vi "Scan Initilize_ver2_2.vi"(0 "VISA Refnum in":refnum<visa-resource-name>, 1 "Scan Measure\nTime":dbl=17.0, 5 "Channel Count":i32, 9 "Current Setting":u8[](array[numeric]), 11 "error in (no error)":errorcluster, 12 "Sample number":i32=1, 13 "Measure Maximun Voltage":dbl=100.0 format="%#_13g", 14 "Enable DMM Relay":bool=TRUE) -> (3 "Current Channel":string[](array[string]), 4 "VISA Refnum out":refnum<visa-resource-name>, 6 "P channel number":i32, 10 "N channel number":i32, 15 "error out":errorcluster)   [LabVIEW 2023]
uses:
  <instrlib>/Agilent 3446X Series/Agilent 3446X Series.lvlib
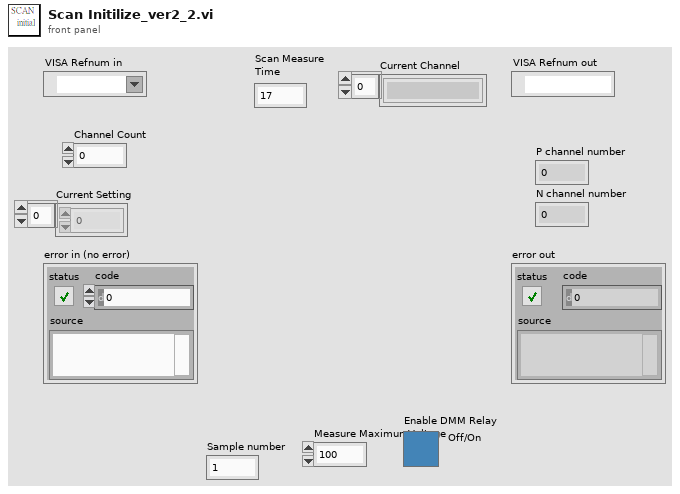
[diagram p1: front panel]
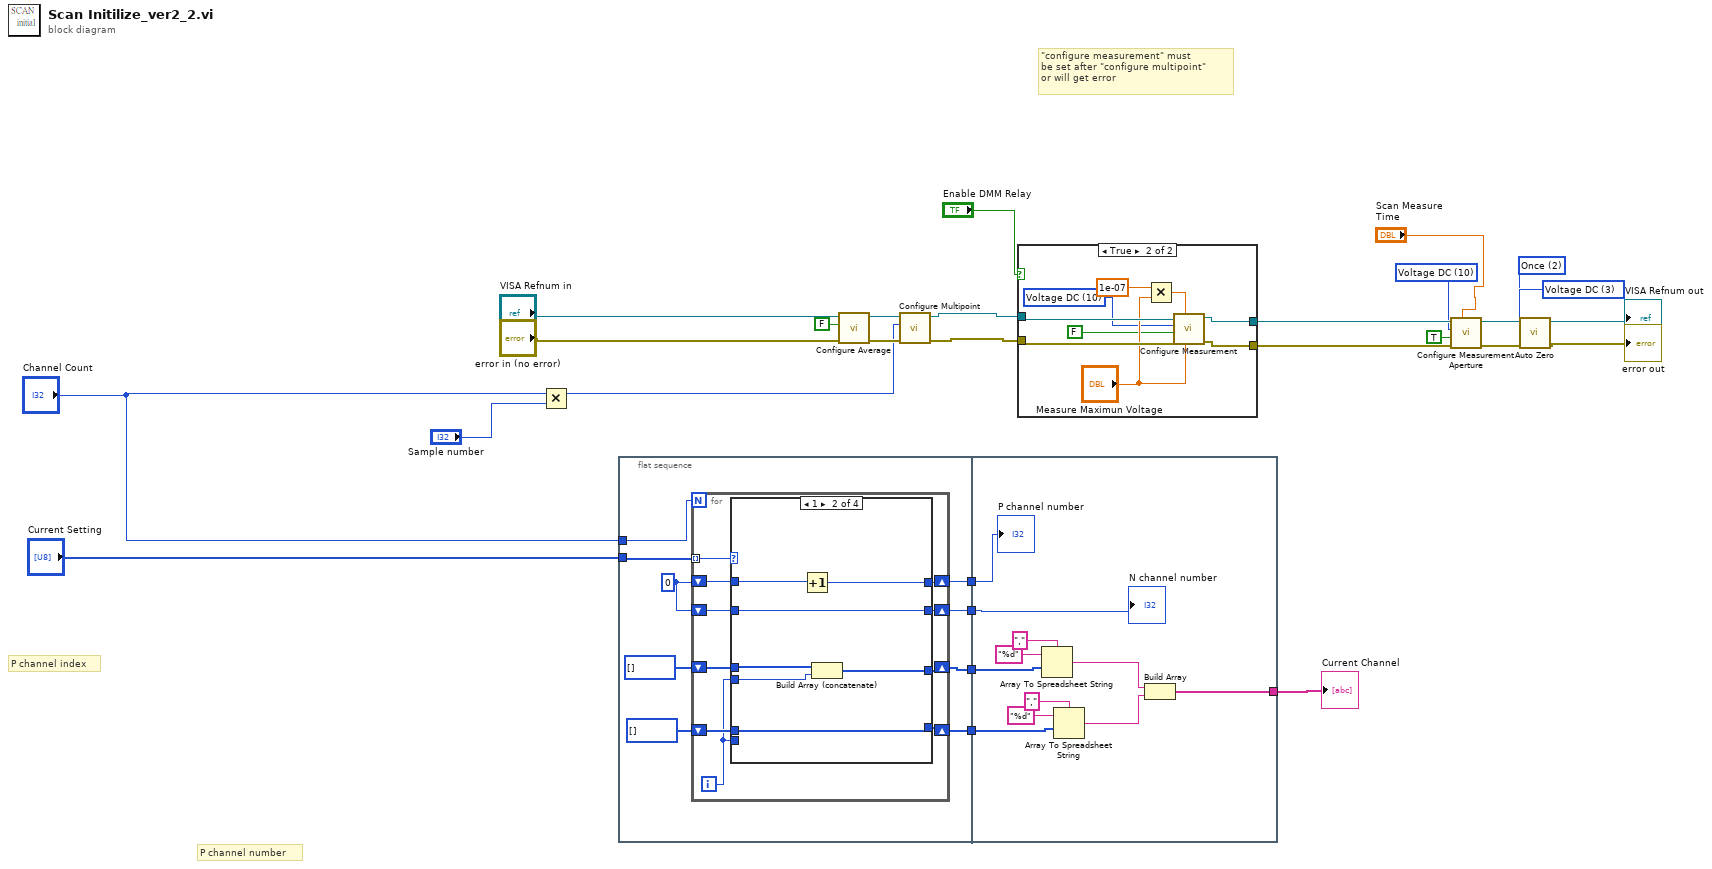
[diagram p0: block diagram]
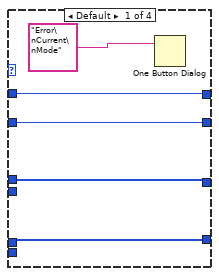
[diagram p3: hidden frame]
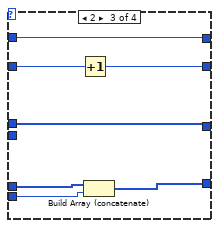
[diagram p4: hidden frame]
diagram:
  w17 = 3 items=["Current DC", "Resistance", "Temperature", "Voltage DC"] ("Zero Type (0: Current DC)")
  w16 = 2 items=["Disable", "Enable", "Once"] ("Auto Zero (1: Enable)")
  w14 = 10 items=["Continuity", "Current AC", "Current DC", "Diode", "Frequency", "Resistance 4-wire", "Period", "Resistance 2-wire", "Temperature", "Voltage AC", "Voltage DC", "Voltage DC Ratio", "Capacitance"] ("Measurement Function (0: Continuity)")
  # "P channel index"
  # "P channel number"
  # "\"configure measurement\" must \nbe set after \"configure multipoint\"\nor will get error"
  n1 = Multiply(x="Channel Count", y="Sample number") -> (x*y=w2:i32)
  n2 = flat-sequence {
    tunnel: "Channel Count" -> [w37]
    tunnel: "Current Setting" -> [w36]
    tunnel: [w34] -> w12
    tunnel: [w33] -> w11
    tunnel: [w30] -> w8
    tunnel: [w29] -> w7
    tunnel: w12 -> [w81]
    tunnel: w11 -> [w80]
    tunnel: w8 -> [w77]
    tunnel: w7 -> [w74]
    tunnel: [w71] -> w6
    frame #0 {
      w35 = 0 ("P_current_count")
      n3 = for {
        N: w37 -> [_]
        tunnel: w36 -> [w47] mode=indexing
        shift-right: [w45] -> w34
        shift-left: w35 -> [w46]
        shift-right: [w43] -> w33
        shift-left: w35 -> [w44]
        shift-right: [w41] -> w30
        shift-left: i32[] [] -> [w42]
        shift-right: [w39] -> w29
        shift-left: i32[] [] -> [w40]
        i -> [w38]
        n4 = case shown="1" w47 {
          tunnel: w46 -> [w51 w59 w64 w70]
          tunnel: [w51 w58 w64 w70] -> w45
          tunnel: w44 -> [w50 w57 w66 w69]
          tunnel: [w50 w57 w65 w69] -> w43
          tunnel: w42 -> [w48 w56 w60 w68]
          tunnel: w38 -> [_ w55 _ _]
          tunnel: [w48 w54 w60 w68] -> w41
          tunnel: w40 -> [w49 w53 w63 w67]
          tunnel: [w49 w53 w62 w67] -> w39
          tunnel: w38 -> [_ _ w61 _]
          frame Default {
            n5 = One Button Dialog(message="Error\nCurrent\nMode" ("error source (\" \")")) -> ()  [unwired: 1 in, 1 out]
          }
          frame 1 {
            n6 = Increment(x=w59) -> (x+1=w58:i32)
            n7 = Build Array (concatenate)(w56, w55) -> (w54:i32[])
          }
          frame 2 {
            n8 = Increment(x=w66) -> (x+1=w65:i32)
            n9 = Build Array (concatenate)(w63, w61) -> (w62:i32[])
          }
          frame 0 {
          }
        }
      }
    }
    frame #1 {
      n10 = Array To Spreadsheet String(delimiter (Tab)=",", array=w77, 3:"%d" ("format string")) -> (spreadsheet string=w73:string)
      n11 = Array To Spreadsheet String(delimiter (Tab)=",", array=w74, 3:"%d" ("format string")) -> (spreadsheet string=w72:string)
      n12 = Build Array(w73, w72) -> (w71:string[])
      "P channel number" <- w81
      "N channel number" <- w80
    }
  }
  n13 = call <instrlib>:"Configure Average.vi"("error in (no error)"="error in (no error)", "Enable Statistics (F: Disable)"=FALSE, "VISA resource name"="VISA Refnum in") -> ("error out"=w22:errorcluster, "VISA resource name out"=w21:refnum<visa-resource-name>)  [unwired: 7 in]
  n14 = call <instrlib>:"Configure Multipoint.vi"("error in (no error)"=w22, "Trigger Count (1)"=w2, "VISA resource name"=w21) -> ("error out"=w24:errorcluster, "VISA resource name out"=w23:refnum<visa-resource-name>)  [unwired: 4 in, 3 out]
  n15 = case shown="True" "Enable DMM Relay" {
    tunnel: [w82 w92] -> w26
    tunnel: [w83 w91] -> w25
    tunnel: w24 -> [w82 w90]
    tunnel: w23 -> [w83 w89]
    frame False {
    }
    frame True {
      w85 = 10 items=["Continuity", "Current AC", "Current DC", "Diode", "Frequency", "Resistance 4-wire", "Period", "Resistance 2-wire", "Temperature", "Voltage AC", "Voltage DC", "Voltage DC Ratio", "Capacitance"] ("Measurement Function (10: Voltage DC)")
      n16 = Multiply(x=1e-07, y="Measure Maximun Voltage") -> (x*y=w86:dbl)
      n17 = call <instrlib>:"Configure Measurement.vi"("Manual Range (1)"="Measure Maximun Voltage", "Absolute Resolution (1E-6)"=w86, "error in (no error)"=w90, "Auto Range (T: Enable)"=FALSE, "Measurement Function (10: Voltage DC)"=w85, "VISA resource name"=w89) -> ("error out"=w92:errorcluster, "VISA resource name out"=w91:refnum<visa-resource-name>)  [unwired: 4 out]
    }
  }
  n18 = call <instrlib>:"Configure Measurement Aperture.vi"("Aperture Time (0.1s)"="Scan Measure\nTime", "error in (no error)"=w26, "Enable Aperture (F: Disable)"=TRUE, "Measurement Function (0: Continuity)"=w14, "VISA resource name"=w25) -> ("error out"=w18:errorcluster, "VISA resource name out"=w20:refnum<visa-resource-name>)  [unwired: 5 in]
  n19 = call <instrlib>:"Auto Zero.vi"("error in (no error)"=w18, "Auto Zero (1: Enable)"=w16, "Zero Type (0: Current DC)"=w17, "VISA resource name"=w20) -> ("error out"=→"error out":errorcluster, "VISA resource name out"=→"VISA Refnum out":refnum<visa-resource-name>)  [unwired: 6 in]
  "Current Channel" <- w6
